vi "Export single dat - CV cluster.vi"(4 ".myDLTS file path":path=path "", 5 "Error In":errorcluster, 6 "Workspace":path, 8 "CV measurement":T1={"Name"="", "Comment"="", "Time"=timestamp(0 s since 1904-01-01), "Folder"=path "", "CV properties"={"T"=0.0, "Vstart"=-0.5, "Vstop"=0.5, "Vpoints"=10.0, "Precision"=enum."Normal", "Test signal"=0.01, "Auto I range"=FALSE, "Test frequency"=100000.0, "I range"=-2.0, "V range"=10.0, "Log mapping"=FALSE, "Rel perm"=0.0, "Area"=0.0}, "GUID"=""} {"CV properties"."V range" items=["10mV"=0.01, "100mV"=0.1, "1V"=1.0, "10V"=10.0]; "CV properties"."I range" items=["100nA"=-7.0, "1µA"=-6.0, "10µA"=-5.0, "100µA"=-4.0, "1mA"=-3.0, "10mA"=-2.0]}) -> (0 "Error Out":errorcluster)   [LabVIEW 2019]
doc: "Handles export of measurement (identified by a tag) to a .dat file, displays a GUI window"
uses:
  Type defs/CV measurement Type Def.ctl
  Type defs/CV properties Type Def.ctl
  <vilib>/Utility/sysdir.llb/System Directory Type.ctl
  <vilib>/Utility/file.llb/Write Delimited Spreadsheet (string).vi
  <vilib>/Utility/file.llb/Write Delimited Spreadsheet (DBL).vi
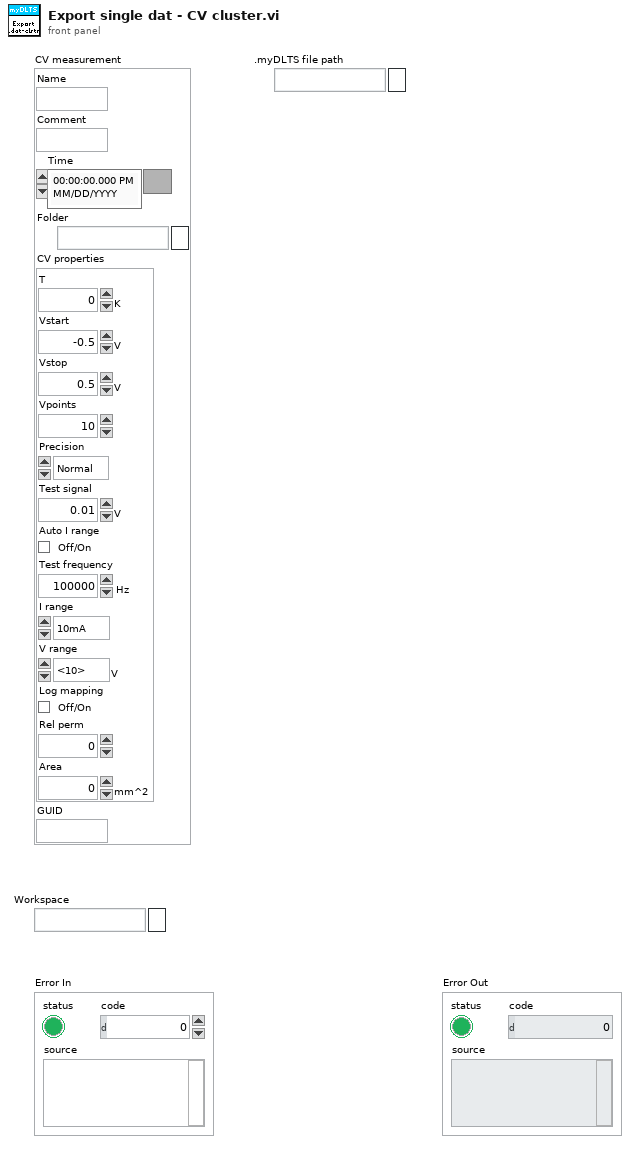
[diagram p1: front panel]
types:
  T1 = typedef "CV measurement Type Def.ctl" = cluster{"Name":string, "Comment":string, "Time":timestamp, "Folder":path, "CV properties":T2, "GUID":string}
  T2 = typedef "CV properties Type Def.ctl" = cluster{"T":dbl[unit], "Vstart":dbl[unit], "Vstop":dbl[unit], "Vpoints":dbl, "Precision":enum16{"Low (Fast)", "Normal", "High (Slow)"}, "Test signal":dbl[unit], "Auto I range":bool, "Test frequency":dbl[unit], "I range":dbl, "V range":dbl[unit], "Log mapping":bool, "Rel perm":dbl, "Area":dbl[unit]}
  T3 = cluster{"Name":string, "Files":path[], "Header":string[][]}
  T4 = typedef "System Directory Type.ctl" = i32
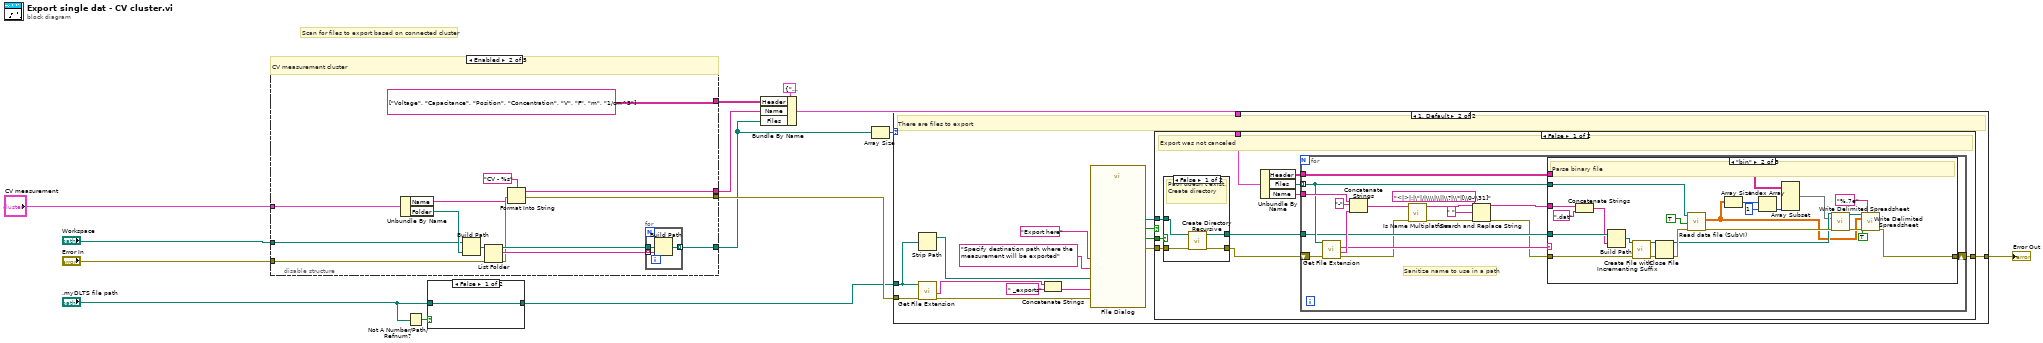
[diagram p0: block diagram]
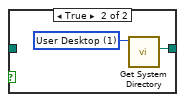
[diagram p2: hidden frame]
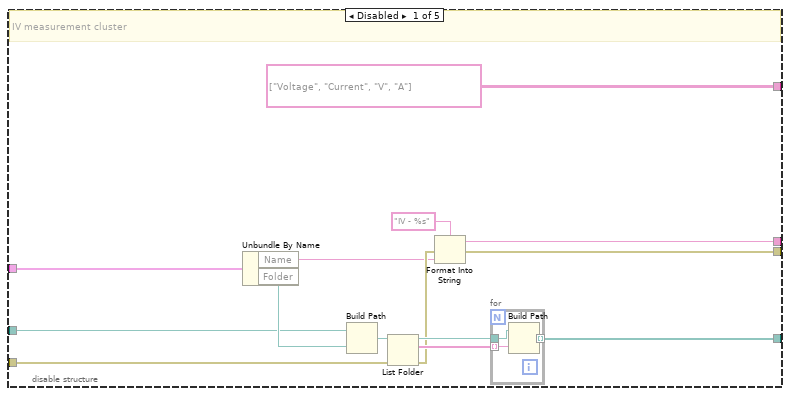
[diagram p3: hidden frame]
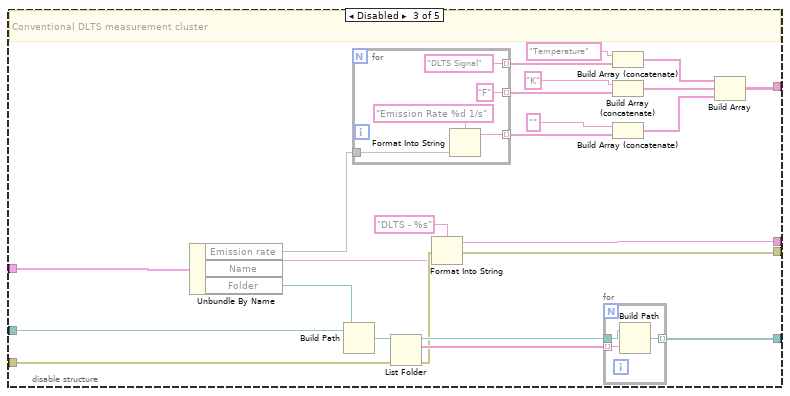
[diagram p4: hidden frame]
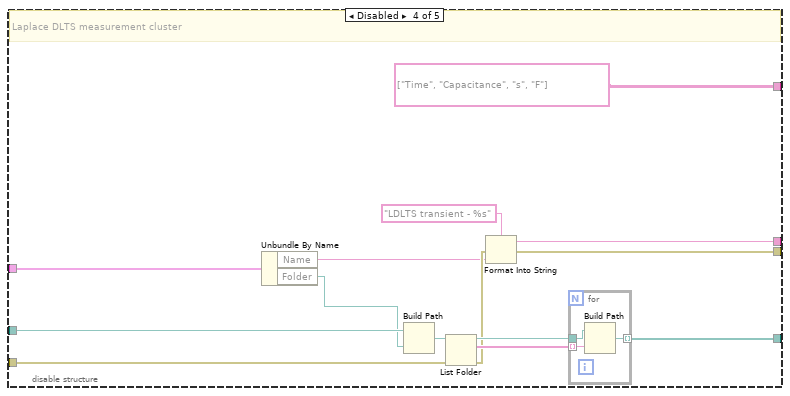
[diagram p5: hidden frame]
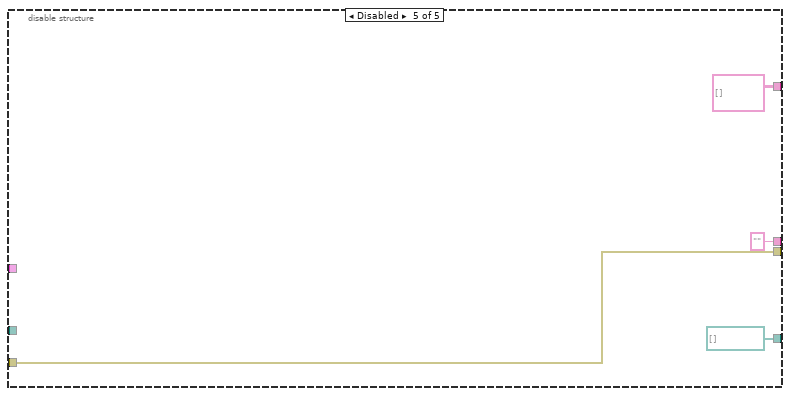
[diagram p6: hidden frame]
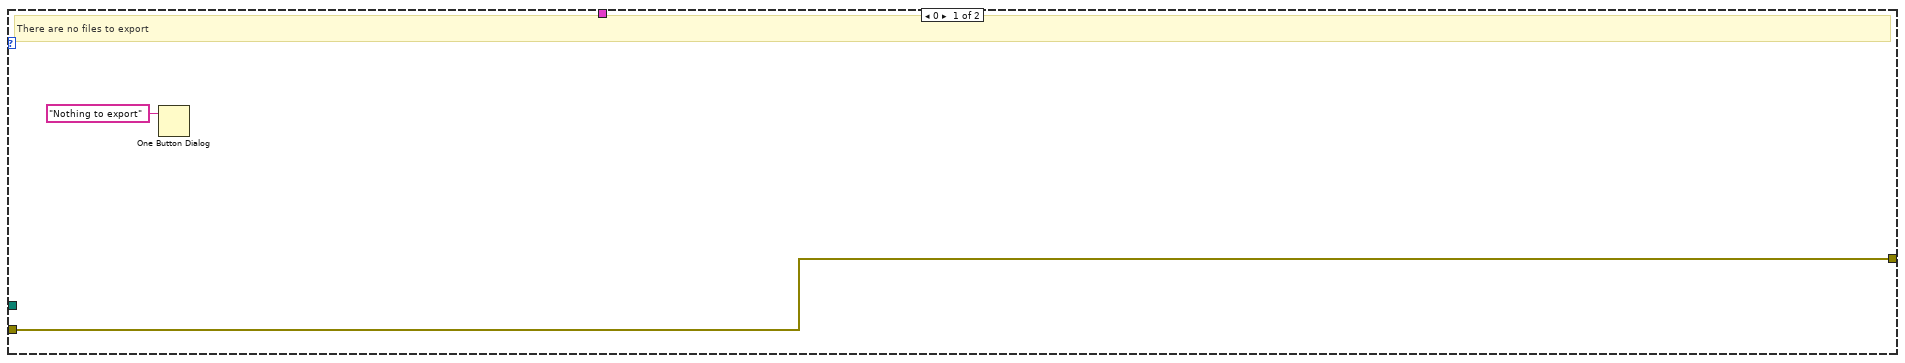
[diagram p7: hidden frame]
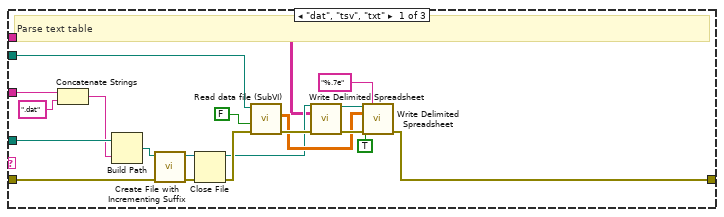
[diagram p8: hidden frame]
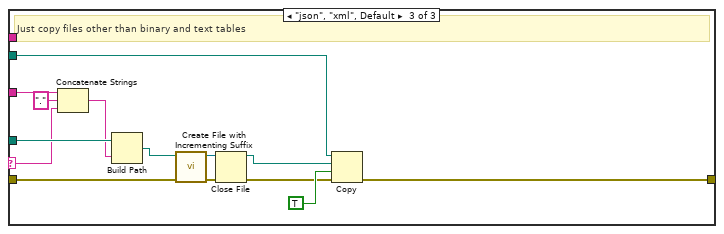
[diagram p9: hidden frame]
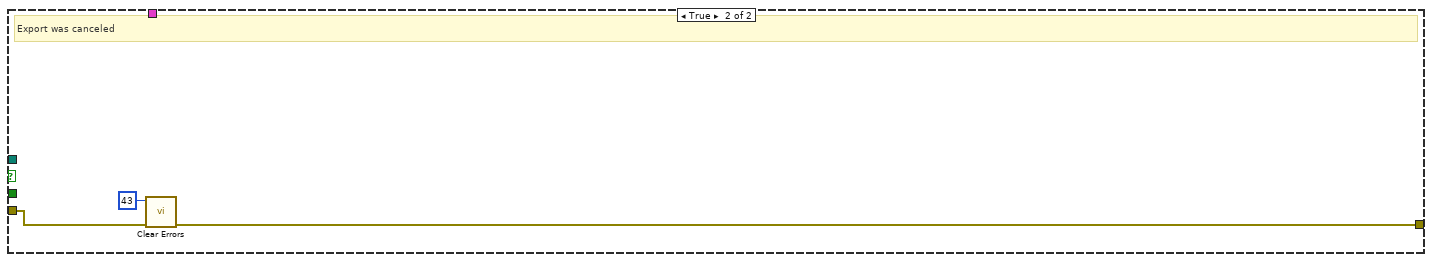
[diagram p11: hidden frame]
diagram:
  # "Scan for files to export based on connected cluster"
  n1 = disable-structure shown="Enabled" {
    disable-tunnel: [string[][] [["Voltage", "Current"], ["V", "A"]] string[][] [["Voltage", "Capacitance", "Position", "Concentration"], ["V", "F", "m", "1/cm^3"]] w55 string[][] [["Time", "Capacitance"], ["s", "F"]] string[][] []] -> w9
    disable-tunnel: [w20 w38 w54 w87 ""] -> w8
    disable-tunnel: [w19 w37 w53 w86 w99] -> w6
    disable-tunnel: [w18 w36 w52 w85 path[] []] -> w5
    disable-tunnel: "Workspace" -> [w17 w34 w50 w83 _]
    disable-tunnel: "Error In" -> [w16 w35 w51 w84 w99]
    disable-tunnel: "CV measurement" -> [w15 w33 w49 w81 _]
    frame Disabled {
      # "IV measurement cluster"
      n2 = Unbundle By Name(w15) -> ("Name"=w22:string, "Folder"=w27:path)
      n3 = Build Path(base path=w17, name or relative path=w27) -> (appended path=w25:path)
      n4 = List Folder(path=w25, error in=w16) -> (path out=w24:path, filenames=w26:string[], error out=w23:errorcluster)  [unwired: 2 in, 1 out]
      n5 = Format Into String(format string="IV - %s", error in=w23, w22) -> (resulting string=w20:string, error out=w19:errorcluster)  [unwired: 1 in]
      n6 = for {
        tunnel: w24 -> [w31]
        tunnel: [w30] -> w18 mode=indexing
        tunnel: w26 -> [w29] mode=indexing
        n7 = Build Path(base path=w31, name or relative path=w29) -> (appended path=w30:path)
      }
    }
    frame Enabled {
      # "CV measurement cluster"
      n8 = Unbundle By Name(w33) -> ("Name"=w39:string, "Folder"=w44:path)
      n9 = Build Path(base path=w34, name or relative path=w44) -> (appended path=w42:path)
      n10 = List Folder(path=w42, error in=w35) -> (path out=w41:path, filenames=w43:string[], error out=w40:errorcluster)  [unwired: 2 in, 1 out]
      n11 = Format Into String(format string="CV - %s", error in=w40, w39) -> (resulting string=w38:string, error out=w37:errorcluster)  [unwired: 1 in]
      n12 = for {
        tunnel: w41 -> [w48]
        tunnel: [w47] -> w36 mode=indexing
        tunnel: w43 -> [w46] mode=indexing
        n13 = Build Path(base path=w48, name or relative path=w46) -> (appended path=w47:path)
      }
    }
    frame Disabled {
      # "Conventional DLTS measurement cluster"
      n14 = Unbundle By Name(w49) -> ("Emission rate"=w57, "Name"=w56:string, "Folder"=w58:path)
      n15 = Build Path(base path=w50, name or relative path=w58) -> (appended path=w69:path)
      n16 = for {
        tunnel: w57 -> [w77]
        tunnel: [w75] -> w64 mode=indexing
        tunnel: ["DLTS Signal"] -> w62 mode=indexing
        tunnel: ["F"] -> w63 mode=indexing
        n17 = Format Into String(format string="Emission Rate %d 1/s", w77) -> (resulting string=w75:string)  [unwired: 2 in, 1 out]
      }
      n18 = List Folder(path=w69, error in=w51) -> (path out=w70:path, filenames=w71:string[], error out=w68:errorcluster)  [unwired: 2 in, 1 out]
      n19 = Format Into String(format string="DLTS - %s", error in=w68, w56) -> (resulting string=w54:string, error out=w53:errorcluster)  [unwired: 1 in]
      n20 = for {
        tunnel: w70 -> [w80]
        tunnel: [w79] -> w52 mode=indexing
        tunnel: w71 -> [w78] mode=indexing
        n21 = Build Path(base path=w80, name or relative path=w78) -> (appended path=w79:path)
      }
      n22 = Build Array (concatenate)("Temperature", w62) -> (w59:string[])
      n23 = Build Array (concatenate)("K", w63) -> (w60:string[])
      n24 = Build Array (concatenate)("", w64) -> (w61:string[])
      n25 = Build Array(w59, w60, w61) -> (w55:string[][])
    }
    frame Disabled {
      # "Laplace DLTS measurement cluster"
      n26 = Unbundle By Name(w81) -> ("Name"=w89:string, "Folder"=w82:path)
      n27 = Build Path(base path=w83, name or relative path=w82) -> (appended path=w92:path)
      n28 = List Folder(path=w92, error in=w84) -> (path out=w91:path, filenames=w93:string[], error out=w90:errorcluster)  [unwired: 2 in, 1 out]
      n29 = Format Into String(format string="LDLTS transient - %s", error in=w90, w89) -> (resulting string=w87:string, error out=w86:errorcluster)  [unwired: 1 in]
      n30 = for {
        tunnel: w91 -> [w97]
        tunnel: [w96] -> w85 mode=indexing
        tunnel: w93 -> [w95] mode=indexing
        n31 = Build Path(base path=w97, name or relative path=w95) -> (appended path=w96:path)
      }
    }
    frame Disabled {
    }
  }
  n32 = Not A Number/Path/Refnum?(number/path/refnum=".myDLTS file path") -> (NaN/Path/Refnum?=w4:bool)
  n33 = case shown="False" w4 {
    tunnel: ".myDLTS file path" -> [w102 _]
    tunnel: [w102 w103] -> w2
    frame False {
    }
    frame True {
      w104 = T4 1 items=["User Home"=0, "User Desktop"=1, "User Documents"=2, "User Application Data"=3, "User Preferences"=4, "User Temporary"=5, "Public Documents"=6, "Public Application Data"=7, "Public Preferences"=8, "Public Cache"=13, "System Core Libraries"=9, "System Installed Libraries"=10, "Application Files"=11, "Boot Volume Root"=12] ("system directory type")
      n34 = call <vilib>:"Get System Directory.vi"("system directory type"=w104) -> ("system directory"=w103:path)  [unwired: 10 in]
    }
  }
  n35 = Bundle By Name(cluster=T3 {"Name"="", "Files"=[], "Header"=[]} ("output cluster"), "Header"=w9, "Name"=w8, "Files"=w5) -> (w7:T3)
  n36 = Array Size(array=w5) -> (size(s)=w14:i32)
  n37 = case shown="1, Default" w14 {
    tunnel: w2 -> [_ w114]
    tunnel: w6 -> [w105 w113]
    tunnel: [w105 w107] -> w12
    tunnel: w7 -> [_ w108]
    frame 0 {
      # "There are no files to export"
      n38 = One Button Dialog(message="Nothing to export") -> ()  [unwired: 1 in, 1 out]
    }
    frame 1, Default {
      # "There are files to export"
      n39 = call <vilib>:"Get File Extension.vi"("error in (no error)"=w113, "file"=w114) -> ("error out"=w118:errorcluster, "filename without extension"=w120:string)  [unwired: 5 in, 3 out]
      n40 = Strip Path(path=w114) -> (stripped path=w119:path)  [unwired: 1 out]
      n41 = Concatenate Strings(w120, " _exports" ("string")) -> (w121:string)
      n42 = call "File Dialog"("start path"=w119, "prompt"="Specify destination path where the measurement will be exported", "button label"="Export here", "default name"=w121, "error in"=w118) -> ("selected path"=w109:path, "exists"=w111:bool, "cancelled"=w112:bool, "error out"=w110:errorcluster)  [unwired: 7 in]
      n43 = case shown="False" w112 {
        tunnel: w111 -> [w131 _]
        tunnel: w110 -> [w130 w215]
        tunnel: w109 -> [w129 _]
        tunnel: w108 -> [w126 _]
        tunnel: [w125 w214] -> w107
        frame False {
          # "Export was not canceled"
          n44 = case shown="False" w131 {
            tunnel: w130 -> [w210 w212]
            tunnel: w129 -> [w209 w211]
            tunnel: [w208 w211] -> w128
            tunnel: [w207 w212] -> w127
            frame False {
              # "Path doesn't exist.\nCreate directory"
              n45 = call <vilib>:"Create Directory Recursive.vi"("error in (no error)"=w210, "directory"=w209) -> ("error out"=w207:errorcluster, "directory copy"=w208:path)  [unwired: 3 in, 1 out]
            }
            frame True {
              # "Path exists"
            }
          }
          n46 = Unbundle By Name(w126) -> ("Header"=w122:string[][], "Files"=w124:path[], "Name"=w123:string)
          n47 = for {
            tunnel: w124 -> [w142] mode=indexing
            tunnel: w123 -> [w147]
            tunnel: w122 -> [w141]
            shift-right: [w143] -> w125
            shift-left: w127 -> [w148]
            tunnel: w128 -> [w140]
            # "Sanitize name to use in a path"
            n48 = call <vilib>:"Get File Extension.vi"("error in (no error)"=w148, "file"=w142) -> ("error out"=w138:errorcluster, "filename without extension"=w145:string, "lowercase file extension"=w144:string)  [unwired: 5 in, 2 out]
            n49 = Concatenate Strings(w147, "-" ("string"), w145) -> (w139:string)
            n50 = call <vilib>:"Is Name Multiplatform.vi"("error in (no error)"=w138, "filename"=w139) -> ("error out"=w134:errorcluster, "suggested filename"=w133:string)  [unwired: 5 in, 3 out]
            n51 = Search and Replace String(input string=w133, search string="<|>|:|\"|/|\\\\|\\||\\?|\\*|[\\0-\\31]", replace string=" " ("replace string (\"\")"), error in=w134) -> (result string=w132:string, error out=w135:errorcluster)  [unwired: 4 in, 2 out]
            n52 = case shown="\"bin\"" w144 {
              selector: w144 -> [_ _ w198]
              tunnel: w132 -> [w168 w192 w206]
              tunnel: w135 -> [w156 w181 w203]
              tunnel: [w155 w180 w193] -> w143
              tunnel: w142 -> [w153 w179 w197]
              tunnel: w141 -> [w154 w170 _]
              tunnel: w140 -> [w151 w177 w202]
              frame "dat", "tsv", "txt" {
                # "Parse text table"
                n53 = Concatenate Strings(w168, ".dat" ("string")) -> (w150:string)
                n54 = Build Path(base path=w151, name or relative path=w150) -> (appended path=w149:path)
                n55 = call <vilib>:"Create File with Incrementing Suffix.vi"("error in (no error)"=w156, "file path"=w149) -> ("error out"=w160:errorcluster, "refnum out"=w159:refnum<file>)  [unwired: 7 in, 1 out]
                n56 = Close File(refnum=w159, error in=w160) -> (path=w157:path, error out=w158:errorcluster)
                n57 = call "Read data file (SubVI).vi"("error in"=w158, "Binary"=FALSE, "file path in"=w153) -> ("error out"=w162:errorcluster, "2D data"=w161:dbl[][])  [unwired: 6 in, 1 out]
                n58 = call-poly <vilib>:"Write Delimited Spreadsheet.vi"("file path (dialog if empty)"=w157, "2D data"=w154, "error in (no error)"=w162) -> ("new file path (Not A Path if cancelled)"=w163:path, "error out"=w165:errorcluster)  [unwired: 11 in]
                n59 = call-poly <vilib>:"Write Delimited Spreadsheet.vi"("file path (dialog if empty)"=w163, "format (%.3f)"="%.7e", "2D data"=w161, "append to file? (new file:F)"=TRUE, "error in (no error)"=w165) -> ("error out"=w155:errorcluster)  [unwired: 9 in, 1 out]
              }
              frame "bin" {
                # "Parse binary file"
                n60 = Concatenate Strings(w192, ".dat" ("string")) -> (w176:string)
                n61 = Build Path(base path=w177, name or relative path=w176) -> (appended path=w175:path)
                n62 = call <vilib>:"Create File with Incrementing Suffix.vi"("error in (no error)"=w181, "file path"=w175) -> ("error out"=w185:errorcluster, "refnum out"=w184:refnum<file>)  [unwired: 7 in, 1 out]
                n63 = Close File(refnum=w184, error in=w185) -> (path=w182:path, error out=w183:errorcluster)
                n64 = call "Read data file (SubVI).vi"("error in"=w183, "Binary"=TRUE, "file path in"=w179) -> ("error out"=w186:errorcluster, "2D data"=w171:dbl[][])  [unwired: 6 in, 1 out]
                n65 = Array Size(array=w171) -> (size(s)=w174:i32[])
                n66 = Index Array(array=w174, index=1) -> (element=w173:i32)
                n67 = Array Subset(array=w170, length (col)=w173) -> (w169:string[][])  [unwired: 3 in]
                n68 = call-poly <vilib>:"Write Delimited Spreadsheet.vi"("file path (dialog if empty)"=w182, "2D data"=w169, "error in (no error)"=w186) -> ("new file path (Not A Path if cancelled)"=w187:path, "error out"=w189:errorcluster)  [unwired: 11 in]
                n69 = call-poly <vilib>:"Write Delimited Spreadsheet.vi"("file path (dialog if empty)"=w187, "format (%.3f)"="%.7e", "2D data"=w171, "append to file? (new file:F)"=TRUE, "error in (no error)"=w189) -> ("error out"=w180:errorcluster)  [unwired: 9 in, 1 out]
              }
              frame "json", "xml", Default {
                # "Just copy files other than binary and text tables"
                n70 = Concatenate Strings(w206, "." ("string"), w198) -> (w201:string)
                n71 = Build Path(base path=w202, name or relative path=w201) -> (appended path=w200:path)
                n72 = call <vilib>:"Create File with Incrementing Suffix.vi"("error in (no error)"=w203, "file path"=w200) -> ("error out"=w205:errorcluster, "refnum out"=w204:refnum<file>)  [unwired: 7 in, 1 out]
                n73 = Close File(refnum=w204, error in=w205) -> (path=w194:path, error out=w195:errorcluster)
                n74 = Copy(8:w195, 9:TRUE ("overwrite (F)"), 10:w194, 11:w197) -> (0:w193:errorcluster)  [unwired: 1 in, 2 out]
              }
            }
          }
        }
        frame True {
          # "Export was canceled"
          n75 = call <vilib>:"Clear Errors.vi"("error in (no error)"=w215, "specific error code to clear (0: all)"=43) -> ("error out"=w214:errorcluster)  [unwired: 4 in, 1 out]
        }
      }
    }
  }
  "Error Out" <- w12
